vi "Action Update Heater State-with-queue-teardown.vi"(8 "error in (no error)":errorcluster) -> (3 "result":bool)   [LabVIEW 2018]
uses:
  Libraries/Thermal Chamber Response Simulator/Thermal Chamber Response Simulator.lvlib
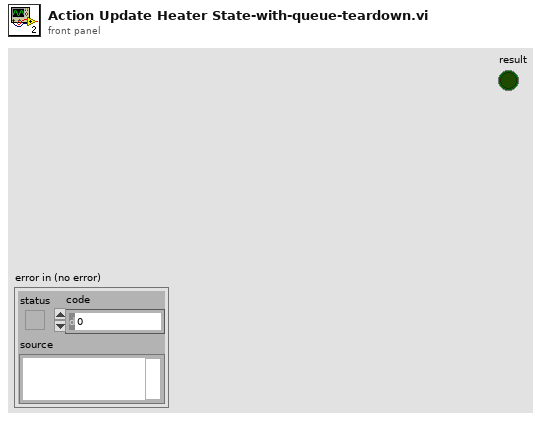
[diagram p1: front panel]
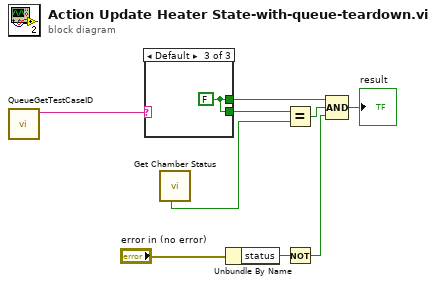
[diagram p0: block diagram]
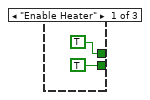
[diagram p2: hidden frame]
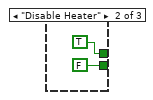
[diagram p3: hidden frame]
diagram:
  n1 = call "QueueGetTestCaseID.vi"() -> ("test case ID"=w1:string)  [unwired: 11 in]
  n2 = case shown="Default" w1 {
    tunnel: [TRUE ("Heater State") FALSE ("Heater State") w14] -> w7
    tunnel: [TRUE ("value") TRUE ("value") w14] -> w5
    frame "Enable Heater" {
    }
    frame "Disable Heater" {
    }
    frame Default {
      w14 = FALSE ("value")
    }
  }
  n3 = call "Get Chamber Status.vi"() -> ("Heater State"=w6:bool)  [unwired: 6 in, 5 out]
  n4 = Unbundle By Name("error in (no error)") -> ("status"=w3:bool)
  n5 = Equal?(x=w7, y=w6) -> (x = y?=w9:bool)
  n6 = Not(x=w3) -> (.not. x?=w2:bool)
  n7 = Compound Arithmetic op=AND(w5, w9, w2) -> (→"result":bool)
